vi "CreateChannel.vi"(8 "error in":errorcluster, 9 "instance":u8, 10 "Channel Info":T1=[{"Channel Name"="Untitled", "Sensitivity mV_EU"=1000.0, "EU"="V", "dB Ref EU"=1.0}, {"Channel Name"="Untitled", "Sensitivity mV_EU"=1000.0, "EU"="V", "dB Ref EU"=1.0}, {"Channel Name"="Untitled", "Sensitivity mV_EU"=1000.0, "EU"="V", "dB Ref EU"=1.0}, {"Channel Name"="Untitled", "Sensitivity mV_EU"=1000.0, "EU"="V", "dB Ref EU"=1.0}] {"dB Ref EU" format="%#.2p"; "Sensitivity mV_EU" format="%.2f"}, 11 "task in":refnum<class "WaveformTask.lvclass">) -> (0 "error out":errorcluster, 3 "Task out":refnum<class "WaveformTask.lvclass">)   [LabVIEW 2015, in "WaveformTask.lvclass"]
uses:
  WaveformTask.lvclass
  <vilib>/NI/cRIO Wfm/ChannelConfig.ctl
  WaveformTask.lvclass/WaveformTask.ctl
  <vilib>/NI/cRIO Wfm/SamplingInfo.ctl
  <instrlib>/_niInstr/Instruction Framework/v1/Host/Subsystem Map/Private/Lookup Single Context.vi
  <vilib>/NI/cRIO Wfm/cRIO Wfm.lvlib
  <instrlib>/_niInstr/Instruction Framework/v1/Host/Subsystem Map/niInstr Subsystem Map v1 Host.lvclass
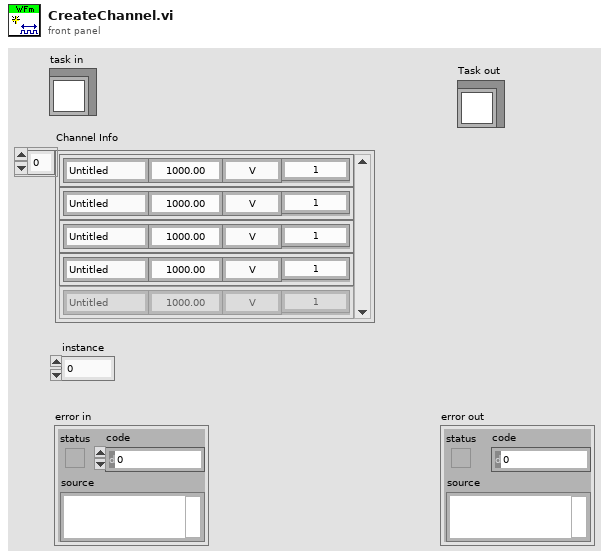
[diagram p1: front panel]
types:
  T1 = typedef "cRIO Wfm.lvlib/ChannelConfig.ctl" = cluster{"Channel Name":string, "Sensitivity mV_EU":dbl, "EU":string, "dB Ref EU":dbl}[]
  T2 = typedef "cRIO Wfm.lvlib/SamplingInfo.ctl" = cluster{"Number of Channels":i32, "Actual Samp Rate":dbl, "Chan Name Array":string[], "EU Chan Array":string[], "dB Ref Chan Array":dbl[]}
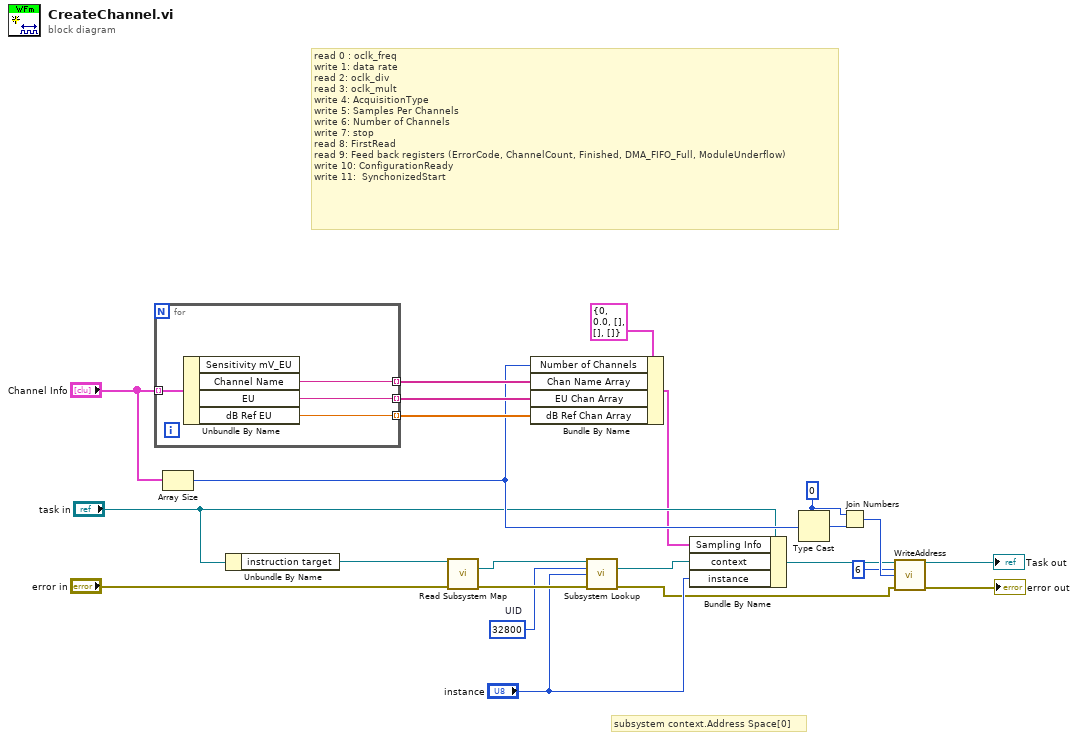
[diagram p0: block diagram]
diagram:
  w13 = u32 0
  w16 = u16 32800  # UID
  # "subsystem context.Address Space[0]"
  # "read 0 : oclk_freq\nwrite 1: data rate\nread 2: oclk_div\nread 3: oclk_mult\nwrite 4: AcquisitionType\nwrite 5: Samples Per Channels\nwrite 6: Number of Channels\nwrite 7: stop\nread 8: FirstRead\nread 9: Feed back registers (ErrorCode, ChannelCount, Finished, DMA_FIFO_Full, ModuleUnderflow)\nwrite 10: ConfigurationReady\nwrite 11:  SynchonizedStart"
  n1 = for {
    tunnel: "Channel Info" -> [w27] mode=indexing
    tunnel: [w25] -> w20 mode=indexing
    tunnel: [w26] -> w21 mode=indexing
    tunnel: [w24] -> w19 mode=indexing
    n2 = Unbundle By Name(w27) -> ("Channel Name"=w24:string, "EU"=w25:string, "dB Ref EU"=w26:dbl)  [unwired: 1 out]
  }
  n3 = Array Size(array="Channel Info") -> (size(s)=w15:i32)
  n4 = Unbundle By Name("task in") -> ("instruction target"=w7:refnum<class "niInstr FIFO Register Bus v1 Host.lvclass">)
  n5 = call <instrlib>:"Read Subsystem Map.vi"("instruction target in"=w7, "error in"="error in") -> ("subsystem map"=w17:refnum<class "niInstr Subsystem Map v1 Host.lvclass">, "error out"=w18:errorcluster)  [unwired: 11 in, 1 out]
  n6 = Bundle By Name(cluster=T2 {"Number of Channels"=0, "Actual Samp Rate"=0.0, "Chan Name Array"=[], "EU Chan Array"=[], "dB Ref Chan Array"=[]} ("Sampling Info"), "Number of Channels"=w15, "Chan Name Array"=w19, "EU Chan Array"=w20, "dB Ref Chan Array"=w21) -> (w1:T2)
  n7 = call-poly <instrlib>:"Subsystem Lookup.vi"("subsystem map in"=w17, "UID"=w16, "instance"="instance", "error in"=w18) -> ("context"=w5:refnum<class "niInstr Instruction Framework Context v1 Host.lvclass">, "error out"=w2:errorcluster)  [unwired: 8 in, 2 out]
  n8 = Bundle By Name(cluster="task in", "Sampling Info"=w1, "context"=w5, "instance"="instance") -> (w3:refnum<class "WaveformTask.lvclass">)
  n9 = Type Cast(type=w13, x=w15) -> (*(type *) &x=w14:u32)
  n10 = Join Numbers(hi=w13, lo=w14) -> ((hi.lo)=w11:u64)
  n11 = call "WriteAddress.vi"("Task in"=w3, "address"=u64 6, "data"=w11, "error in (no error)"=w2) -> ("Task out"=→"Task out":refnum<class "WaveformTask.lvclass">, "error out"=→"error out":errorcluster)  [unwired: 10 in]
